vi "TagDB Read Data Example.vi"() -> ()   [LabVIEW 2017]
uses:
  TagDB Application Example/DEF-SineSettings.ctl
  c988338c-dfcd-45ae-a170-0c12240f6647.vi
  6f91cf01-4a07-448c-baa5-5edfb62a1f80.vi
  0c6764e1-d24c-46ec-b904-80df9fc25c48.vi
  TagDB/_Support/DataAccess/data-Write.vi
  TagDB/_Support/URL/TRIM-BOTH-SPACE.vi
  TagDB/_Support/Error/_[error50000]Invalid DB REF.vi
  TagDB/_Support/DataAccess/TagDB Ref to DVR.vi
  TagDB/_Support/DataAccess/_NameCacher.vi
  TagDB/_Support/Error/_[error50002]Invalid DataType.vi
  TagDB/_Support/DataAccess/_datatypeChecker.vi
  <vilib>/Utility/Data Type/Get Type Information.vi
  TagDB/_Support/Error/_Build Error Cluster.vi
  TagDB/TagDB.lvlib
panel:
  out "Value 2":T1
  out "Value":T2
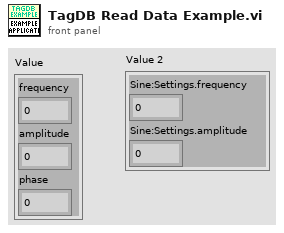
[diagram p1: front panel]
types:
  T1 = cluster{"Sine:Settings.frequency":dbl, "Sine:Settings.amplitude":dbl}
  T2 = cluster{"frequency":dbl, "amplitude":dbl, "phase":dbl}
  T3 = typedef "DEF-SineSettings.ctl" = cluster{"frequency":dbl, "amplitude":dbl, "phase":dbl, "sampling info":cluster{"Fs":dbl, "#s":dbl}}
  T4 = typedef "TagDB.lvlib/TagDB.ctl" = refnum<k1>
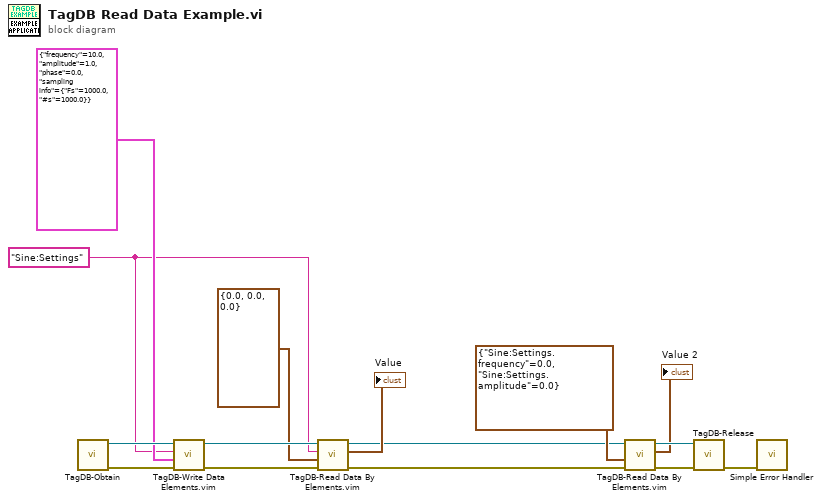
[diagram p0: block diagram]
diagram:
  w9 = "Sine:Settings" ("name")
  n1 = call "TagDB-Obtain.vi"() -> ("error out"=w13:errorcluster, "TagDB"=w14:T4)  [unwired: 5 in, 1 out]
  n2 = call "TagDB-Write Data Elements.vim"("error in (no error)"=w13, "Value"=T3 {"frequency"=10.0, "amplitude"=1.0, "phase"=0.0, "sampling info"={"Fs"=1000.0, "#s"=1000.0}} ("Sine Settings"), "root tag"=w9, "TagDB"=w14) -> ("error out"=w11:errorcluster, "TagDB(dup)"=w10:T4)  [unwired: 5 in, 1 out]
  n3 = call "TagDB-Read Data By Elements.vim"("error in (no error)"=w11, "Type(empty to read as variant)"=T2 {"frequency"=0.0, "amplitude"=0.0, "phase"=0.0} ("Sine Settings"), "Root Tag"=w9, "TagDB"=w10) -> ("error out"=w4:errorcluster, "Value"=→"Value":T2, "TagDB(dup)"=w5:T4)  [unwired: 4 in, 1 out]
  n4 = call "TagDB-Read Data By Elements.vim"("error in (no error)"=w4, "Type(empty to read as variant)"=T1 {"Sine:Settings.frequency"=0.0, "Sine:Settings.amplitude"=0.0} ("Sine Settings"), "TagDB"=w5) -> ("error out"=w3:errorcluster, "Value"=→"Value 2":T1, "TagDB(dup)"=w2:T4)  [unwired: 5 in, 1 out]
  n5 = call "TagDB-Release.vi"("error in (no error)"=w3, "TagDB"=w2) -> ("error out"=w15:errorcluster)  [unwired: 9 in]
  n6 = call <vilib>:"Simple Error Handler.vi"("error in (no error)"=w15) -> ()  [unwired: 4 in, 5 out]
